vi "HDMIDiffractiveTest.vi"() -> ()   [LabVIEW 2010]
uses:
  Program Files/Meadowlark Optics/Blink 1920 HDMI/SDK/Blink_C_wrapper.dll
  <vilib>/Utility/file.llb/Write To Spreadsheet File (I64).vi
  ImageGen.dll
panel:
  out "Array":u8[][](array[numeric])
  # "Load diffraction patterns to the SLM, and measure 1st order intensity to calibrate a LUT\nCan be used to generate a global or regional LUT"
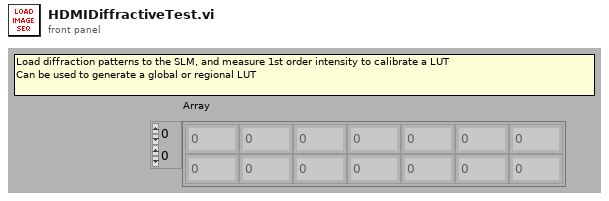
[diagram p1: front panel]
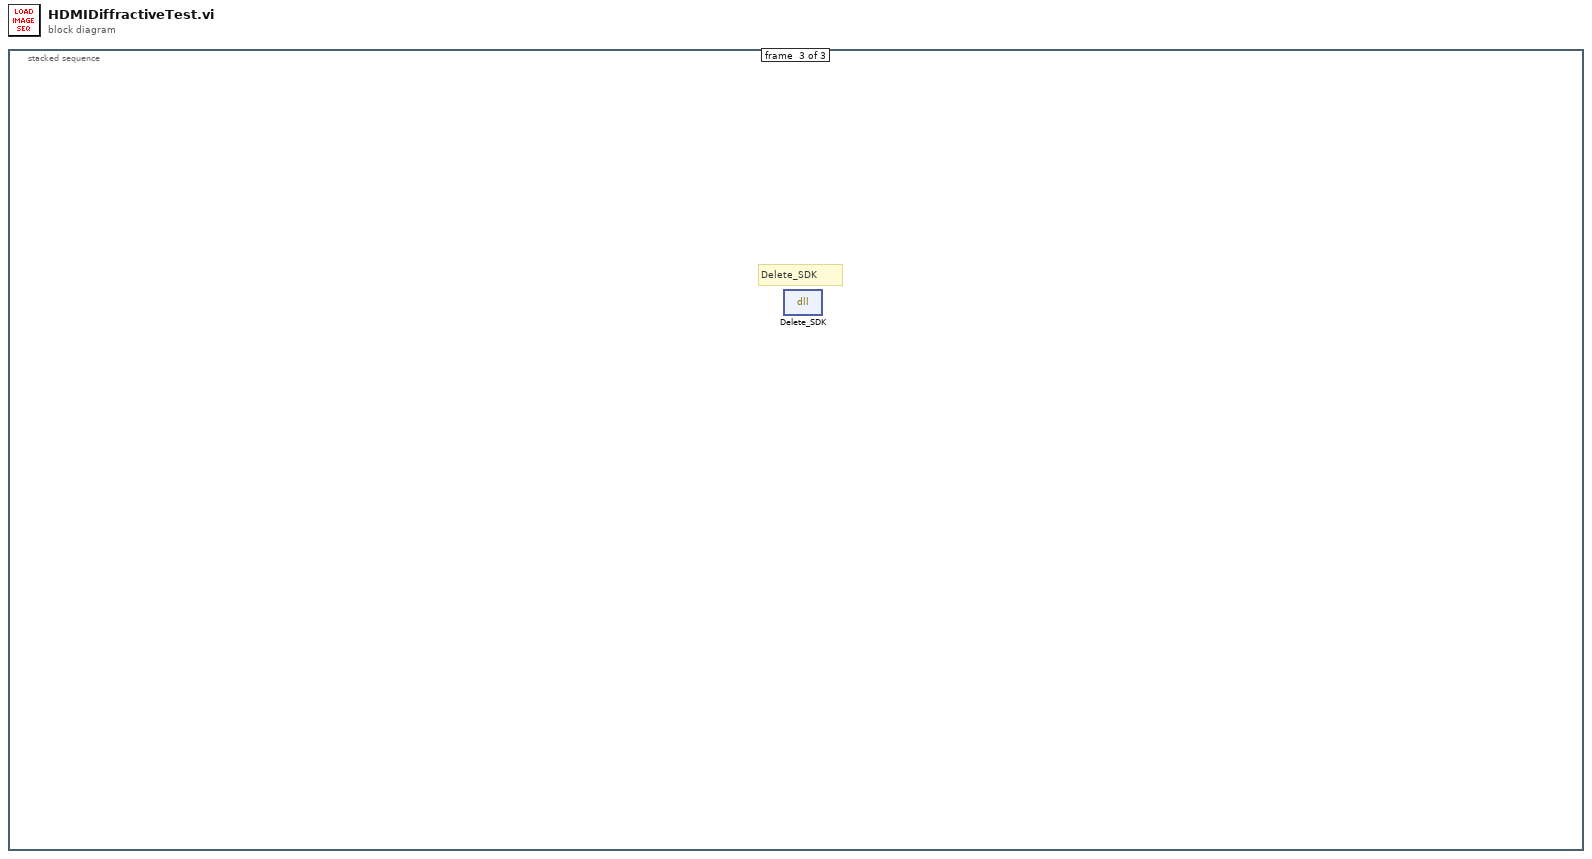
[diagram p0: block diagram]
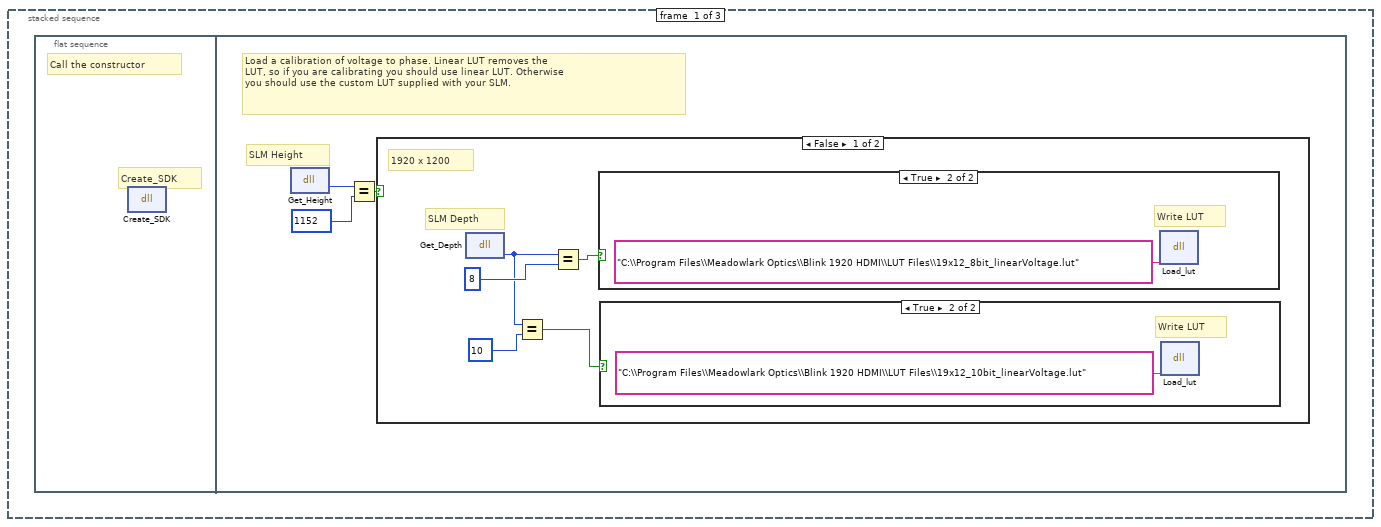
[diagram p2: hidden frame]
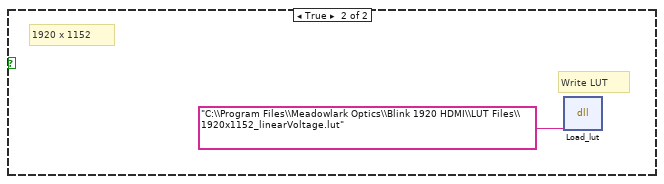
[diagram p5: hidden frame]
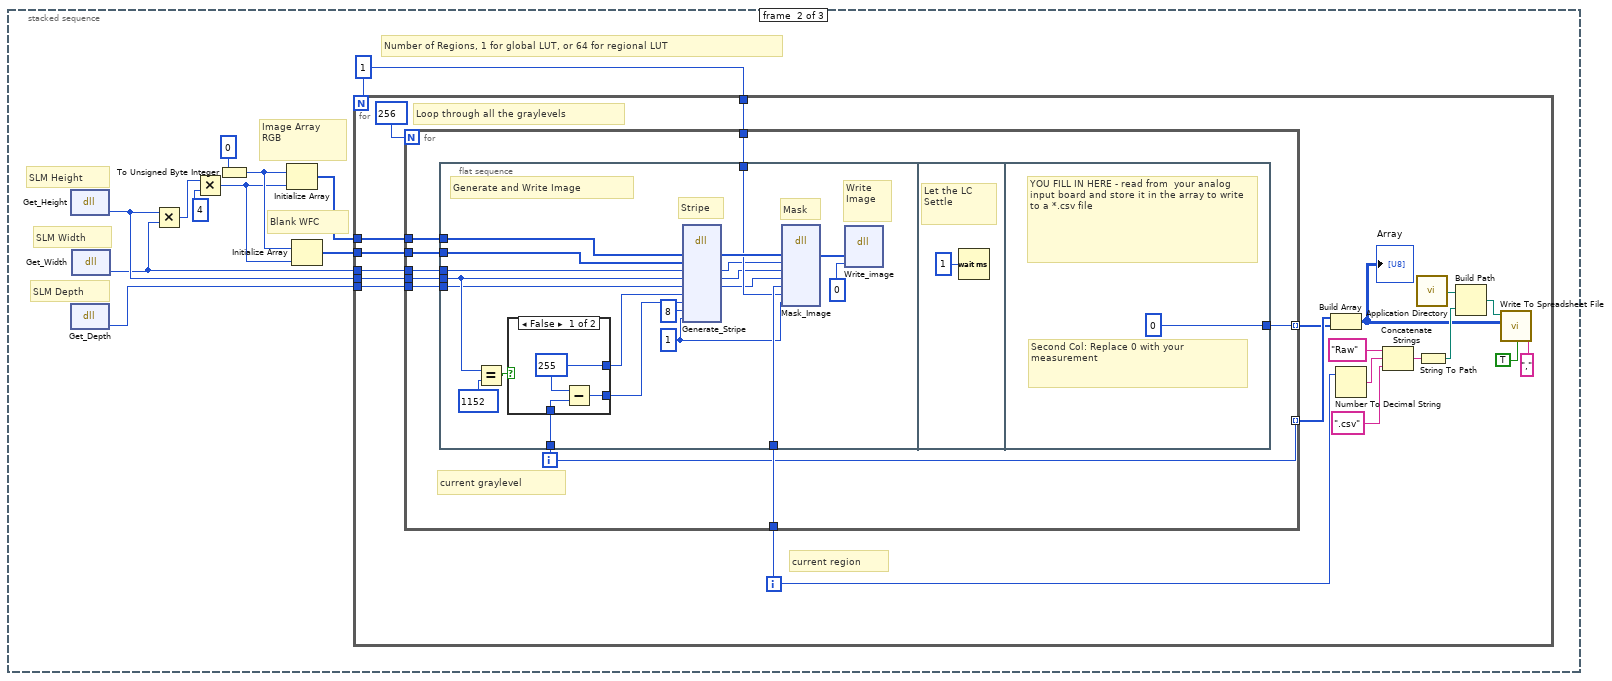
[diagram p6: hidden frame]
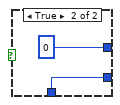
[diagram p7: hidden frame]
diagram:
  n1 = stacked-sequence {
    frame #0 {
      n2 = flat-sequence {
        frame #0 {
          # "Call the constructor"
          # "Create_SDK"
          n3 = dll-call lib="C:/Program Files/Meadowlark Optics/Blink 1920 HDMI/SDK/Blink_C_wrapper.dll" fn="Create_SDK"() -> ()  [unwired: 4 in, 2 out]
        }
        frame #1 {
          # "SLM Height"
          # "Load a calibration of voltage to phase. Linear LUT removes the \nLUT, so if you are calibrating you should use linear LUT. Otherwise \nyou should use the custom LUT supplied with your SLM."
          n4 = dll-call lib="C:/Program Files/Meadowlark Optics/Blink 1920 HDMI/SDK/Blink_C_wrapper.dll" fn="Get_Height"() -> ("return type"=w1:i32)  [unwired: 3 in, 2 out]
          n5 = Equal?(x=w1, y=1152) -> (x = y?=w3:bool)
          n6 = case shown="False" w3 {
            frame False {
              # "1920 x 1200"
              # "SLM Depth"
              n7 = dll-call lib="C:/Program Files/Meadowlark Optics/Blink 1920 HDMI/SDK/Blink_C_wrapper.dll" fn="Get_Depth"() -> ("return type"=w7:i32)  [unwired: 3 in, 2 out]
              n8 = Equal?(x=w7, y=10) -> (x = y?=w5:bool)
              n9 = Equal?(x=w7, y=8) -> (x = y?=w4:bool)
              n10 = case shown="True" w4 {
                frame False {
                }
                frame True {
                  # "Write LUT"
                  n11 = dll-call lib="C:/Program Files/Meadowlark Optics/Blink 1920 HDMI/SDK/Blink_C_wrapper.dll" fn="Load_lut"("Path"="C:\\Program Files\\Meadowlark Optics\\Blink 1920 HDMI\\LUT Files\\19x12_8bit_linearVoltage.lut") -> ()  [unwired: 5 in, 2 out]
                }
              }
              n12 = case shown="True" w5 {
                frame False {
                }
                frame True {
                  # "Write LUT"
                  n13 = dll-call lib="C:/Program Files/Meadowlark Optics/Blink 1920 HDMI/SDK/Blink_C_wrapper.dll" fn="Load_lut"("Path"="C:\\Program Files\\Meadowlark Optics\\Blink 1920 HDMI\\LUT Files\\19x12_10bit_linearVoltage.lut") -> ()  [unwired: 5 in, 2 out]
                }
              }
            }
            frame True {
              # "1920 x 1152"
              # "Write LUT"
              n14 = dll-call lib="C:/Program Files/Meadowlark Optics/Blink 1920 HDMI/SDK/Blink_C_wrapper.dll" fn="Load_lut"("Path"="C:\\Program Files\\Meadowlark Optics\\Blink 1920 HDMI\\LUT Files\\1920x1152_linearVoltage.lut") -> ()  [unwired: 5 in, 2 out]
            }
          }
        }
      }
    }
    frame #1 {
      w20 = 1
      # "Blank WFC"
      # "SLM Depth"
      # "Number of Regions, 1 for global LUT, or 64 for regional LUT"
      # "SLM Width"
      # "SLM Height"
      # "Image Array\nRGB"
      n15 = dll-call lib="C:/Program Files/Meadowlark Optics/Blink 1920 HDMI/SDK/Blink_C_wrapper.dll" fn="Get_Height"() -> ("return type"=w19:i32)  [unwired: 3 in, 2 out]
      n16 = dll-call lib="C:/Program Files/Meadowlark Optics/Blink 1920 HDMI/SDK/Blink_C_wrapper.dll" fn="Get_Depth"() -> ("return type"=w12:i32)  [unwired: 3 in, 2 out]
      n17 = dll-call lib="C:/Program Files/Meadowlark Optics/Blink 1920 HDMI/SDK/Blink_C_wrapper.dll" fn="Get_Width"() -> ("return type"=w18:i32)  [unwired: 3 in, 2 out]
      n18 = Multiply(x=w19, y=w18) -> (x*y=w17:i32)
      n19 = Multiply(x=w17, y=4) -> (x*y=w14:i32)
      n20 = To Unsigned Byte Integer(number=0) -> (unsigned 8bit integer=w15:u8)
      n21 = Initialize Array(w15, w14) -> (w21:u8[])
      n22 = Initialize Array(w15, w14) -> (w13:u8[])
      n23 = for {
        N: w20 -> [_]
        tunnel: w21 -> [w42]
        tunnel: w18 -> [w41]
        tunnel: w19 -> [w40]
        tunnel: w20 -> [w38]
        tunnel: w13 -> [w24]
        tunnel: w12 -> [w23]
        i -> [w36]
        # "Loop through all the graylevels"
        # "current region"
        n24 = for {
          N: 256 -> [_]
          tunnel: w42 -> [w51]
          tunnel: w41 -> [w50]
          tunnel: w40 -> [w49]
          tunnel: w36 -> [w48]
          tunnel: w38 -> [w47]
          tunnel: [w46] -> w26 mode=indexing
          tunnel: [w45] -> w25 mode=indexing
          tunnel: w24 -> [w44]
          tunnel: w23 -> [w43]
          i -> [w46]
          # "current graylevel"
          n25 = flat-sequence {
            tunnel: w51 -> [w71]
            tunnel: w50 -> [w69]
            tunnel: w49 -> [w63]
            tunnel: w48 -> [w66]
            tunnel: w47 -> [w65]
            tunnel: w46 -> [w60]
            tunnel: w44 -> [w57]
            tunnel: w43 -> [w56]
            tunnel: [0] -> w45
            frame #0 {
              w52 = 1
              # "Generate and Write Image"
              # "Write \nImage"
              # "Mask"
              # "Stripe"
              n26 = Equal?(x=w63, y=1152) -> (x = y?=w61:bool)
              n27 = case shown="False" w61 {
                tunnel: w60 -> [w74 w75]
                tunnel: [w73 0] -> w59
                tunnel: [w72 w75] -> w58
                frame False {
                  w73 = 255
                  n28 = Subtract(x=w73, y=w74) -> (x-y=w72:i32)
                }
                frame True {
                }
              }
              n29 = dll-call lib="C:/Meadowlark/Repos-git/MeadowlarkBison/BlinkSdkExample/ImageGen.dll" fn="Generate_Stripe"("Array"=w71, "WFC"=w57, "Width"=w69, "Height"=w63, "Depth"=w56, "PixelValOne"=w59, "PixelValTwo"=w58, "PixelsPerStripe"=8, "RGB"=w52) -> ("Array"=w70:u8[], "Width"=w53:i32, "Height"=w54:i32, "Depth"=w55:i32)  [unwired: 9 in, 2 out]
              n30 = dll-call lib="C:/Meadowlark/Repos-git/MeadowlarkBison/BlinkSdkExample/ImageGen.dll" fn="Mask_Image"("Array"=w70, "Width"=w53, "Height"=w54, "Depth"=w55, "Region"=w66, "NumRegions"=w65, "RGB"=w52) -> ("Array"=w67:u8[])  [unwired: 10 in, 2 out]
              n31 = dll-call lib="C:/Program Files/Meadowlark Optics/Blink 1920 HDMI/SDK/Blink_C_wrapper.dll" fn="Write_image"("image_data"=w67, "isEightBit"=0) -> ()  [unwired: 6 in, 2 out]
            }
            frame #1 {
              # "Let the LC \nSettle"
              n32 = Wait (ms)(milliseconds to wait=u32 1) -> ()  [unwired: 1 out]
            }
            frame #2 {
              # "Second Col: Replace 0 with your measurement"
              # "YOU FILL IN HERE - read from  your analog input board and store it in the array to write to a *.csv file"
            }
          }
        }
        n33 = Build Array(w26, w25) -> (w27:i32[][])
        "Array" <- w27
        n34 = Number To Decimal String(number=w36) -> (decimal integer string=w35:string)  [unwired: 1 in]
        n35 = Concatenate Strings("Raw", w35, ".csv") -> (w33:string)
        n36 = call <vilib>:"Application Directory.vi"() -> ("Application Directory"=w32:path)
        n37 = String To Path(string=w33) -> (path=w31:path)
        n38 = Build Path(base path=w32, name or relative path=w31) -> (appended path=w30:path)
        n39 = call-poly <vilib>:"Write To Spreadsheet File.vi"("delimiter (\\t)"=",", "transpose? (no:F)"=TRUE, "2D data"=w27, "file path (dialog if empty)"=w30) -> ()  [unwired: 4 in, 1 out]
      }
    }
    frame #2 {
      # "Delete_SDK"
      n40 = dll-call lib="C:/Program Files/Meadowlark Optics/Blink 1920 HDMI/SDK/Blink_C_wrapper.dll" fn="Delete_SDK"() -> ()  [unwired: 4 in, 2 out]
    }
  }
